vi "SetupPiplelineChain.vi"(8 "error in (no error)":errorcluster, 9 "Enqueuer":refnum<class "Message Enqueuer.lvclass">, 10 "Destination":string, 11 "Microscope in":refnum<class "Microscope.lvclass">) -> (0 "error out":errorcluster, 1 "Enqueuer dup":refnum<class "Message Enqueuer.lvclass">, 2 "Destination dup":string, 3 "Microscope out":refnum<class "Microscope.lvclass">)   [LabVIEW 2020, in "Microscope.lvlib" / "Microscope.lvclass"]
uses:
  Microscope.lvclass
  <vilib>/ActorFramework/Message Enqueuer/Message Enqueuer.lvclass
  Microscope.lvclass/Microscope.ctl
  Component/Device/Device/DataExchange.ctl
  Interface/DataListener Messages/OnDataChange Msg/OnDataChange Msg.lvclass/OnDataChange Msg.ctl
  <vilib>/ActorFramework/Message Enqueuer/Message Enqueuer.lvclass/Message Enqueuer.ctl
  <vilib>/ActorFramework/Message Enqueuer/Enqueue.vi
  Interface/DataListener Messages/OnDataChange Msg/OnDataChange Msg.lvclass
  C:/Program Files/National Instruments/LabVIEW 2020/vi.lib/ActorFramework/Message/Message.lvclass
  <vilib>/ActorFramework/Message Priority Queue/Priority Enqueue.vi
  Interface/DataListener/DataListener.lvclass
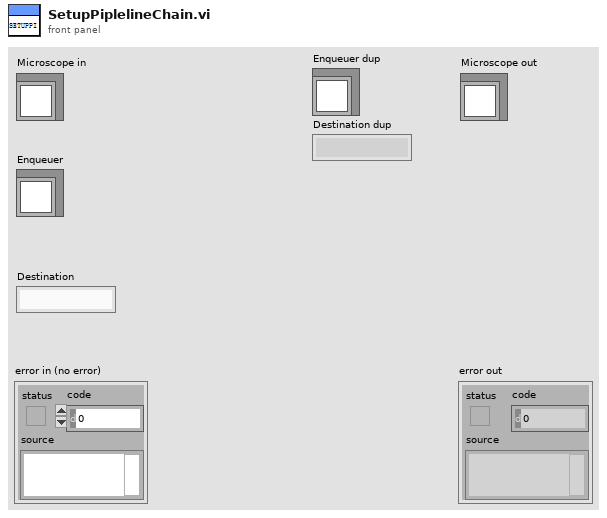
[diagram p1: front panel]
types:
  T1 = typedef "DataListener.lvclass/DataExchange.ctl" = cluster{"Source":string, "Destination":string, "Description":string, "value":variant}
  T2 = cluster{"Enqueuer":refnum<class "Message Enqueuer.lvclass">, "Label":string}
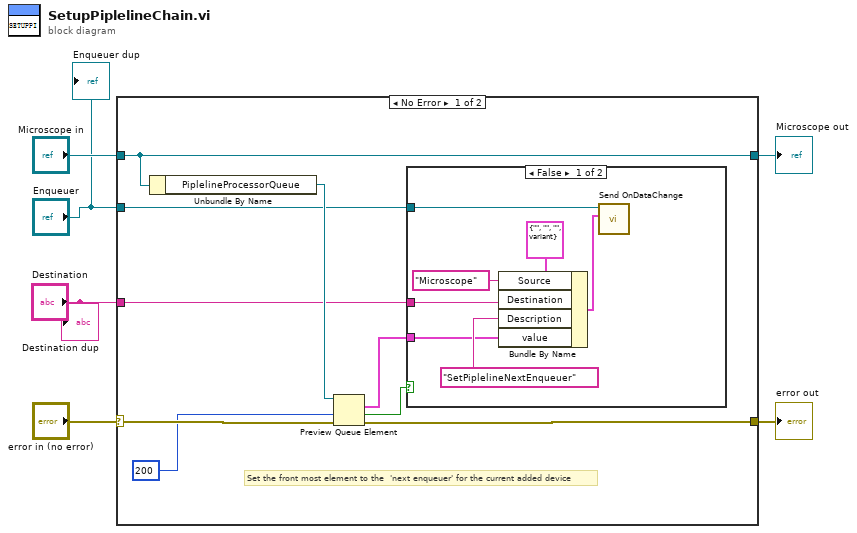
[diagram p0: block diagram]
diagram:
  n1 = case shown="No Error" "error in (no error)" {
    selector: "error in (no error)" -> [w15 w24]
    tunnel: [w13 w24] -> w5
    tunnel: [w14 w23] -> w3
    tunnel: "Microscope in" -> [w14 w23]
    tunnel: "Destination" -> [w8 _]
    tunnel: "Enqueuer" -> [w7 _]
    frame No Error {
      # "Set the front most element to the  'next enqueuer' for the current added device"
      n2 = Unbundle By Name(w14) -> ("PiplelineProcessorQueue"=w12:refnum<queue>)
      n3 = Preview Queue Element(queue=w12, timeout in ms (-1)=200, error in (no error)=w15) -> (element=w9:T2, timed out?=w10:bool, error out=w13:errorcluster)  [unwired: 1 out]
      n4 = case shown="False" w10 {
        tunnel: w9 -> [w19 _]
        tunnel: w8 -> [w18 _]
        tunnel: w7 -> [w17 _]
        frame False {
          n5 = Bundle By Name(cluster=T1 {"Source"="", "Destination"="", "Description"="", "value"=variant} ("DataExchange"), "Source"="Microscope", "Destination"=w18, "Description"="SetPiplelineNextEnqueuer", "value"=w19) -> (w21:T1)
          n6 = call "Send OnDataChange.vi"("DataExchange"=w21, "Message Enqueuer"=w17) -> ()  [unwired: 8 in, 2 out]
        }
        frame True {
        }
      }
    }
    frame Error {
    }
  }
  "error out" <- w5
  "Microscope out" <- w3
  "Enqueuer dup" <- "Enqueuer"
  "Destination dup" <- "Destination"
